vi "PAN_RunAsyncSet.vi"(7 "nodeID":string, 8 "error in (no error)":errorcluster, 10 "msg in":string, 11 "type specifier VI Refnum (for type only)":refnum<vi>) -> (0 "error out":errorcluster, 2 "resp out":string, 3 "reference out":refnum<vi>)   [LabVIEW 2016]
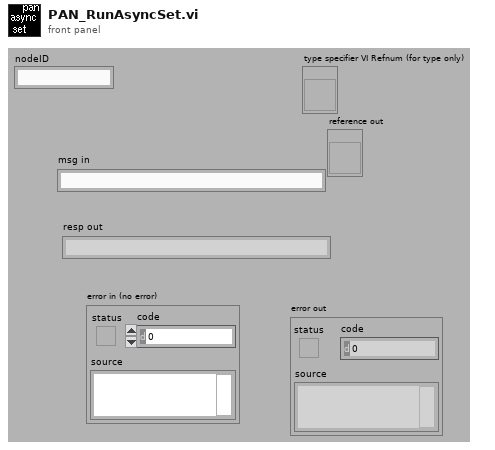
[diagram p1: front panel]
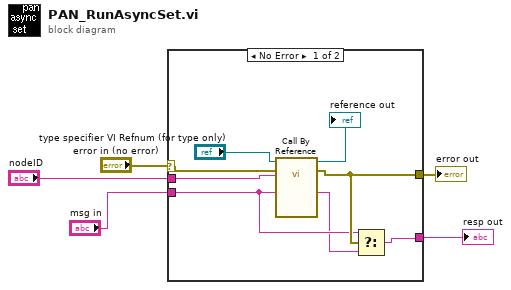
[diagram p0: block diagram]
diagram:
  n1 = case shown="No Error" "error in (no error)" {
    selector: "error in (no error)" -> [w12 w15]
    tunnel: [w10 w15] -> w5
    tunnel: "msg in" -> [w9 w14]
    tunnel: [w7 w14] -> w3
    tunnel: "nodeID" -> [w11 _]
    frame No Error {
      n2 = call-by-ref "?"(reference="type specifier VI Refnum (for type only)", error in=w12, "nodeID"=w11, "msg in"=w9) -> (reference out=→"reference out":refnum<vi>, error out=w10:errorcluster, "msg out"=w8:string)  [unwired: 9 in]
      n3 = Select(t=w9, s=w10, f=w8) -> (s? t:f=w7:string)
    }
    frame Error {
    }
  }
  "error out" <- w5
  "resp out" <- w3
